vi "Do Action.vi"(7 "Self Enqueuer":refnum<class "Message Enqueuer.lvclass">, 8 "error in (no error)":errorcluster, 11 "Show Assert in":refnum<class "Show Assert.lvclass">) -> (0 "error out":errorcluster)   [LabVIEW 2016, in "Assert API Components.lvlib" / "Assert Display.lvlib" / "Main Display.lvlib" / "Show Assert.lvclass"]
uses:
  Show Assert.lvclass
  <vilib>/ActorFramework/Message Enqueuer/Message Enqueuer.lvclass
  <vilib>/Utility/traverseref.llb/TRef TravTarget.ctl
  Show Assert.lvclass/Show Assert.ctl
  Assert API Components/Assert API Components.lvlib
  <vilib>/Utility/traverseref.llb/VI Scripting - Traverse.lvlib
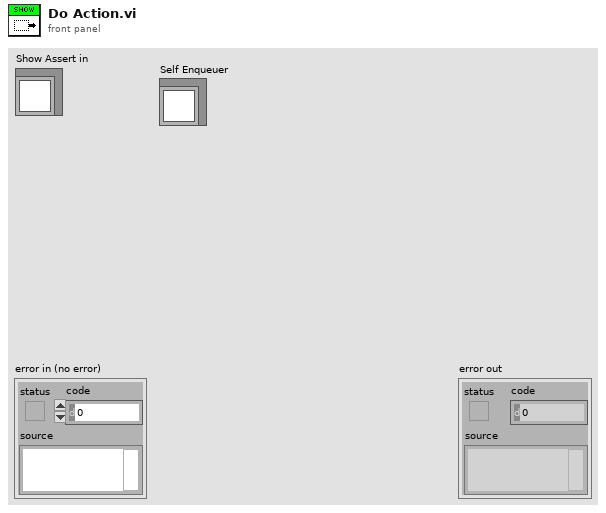
[diagram p1: front panel]
types:
  T1 = typedef "TRef TravTarget.ctl" = enum16{"FP", "BD", "Other"}
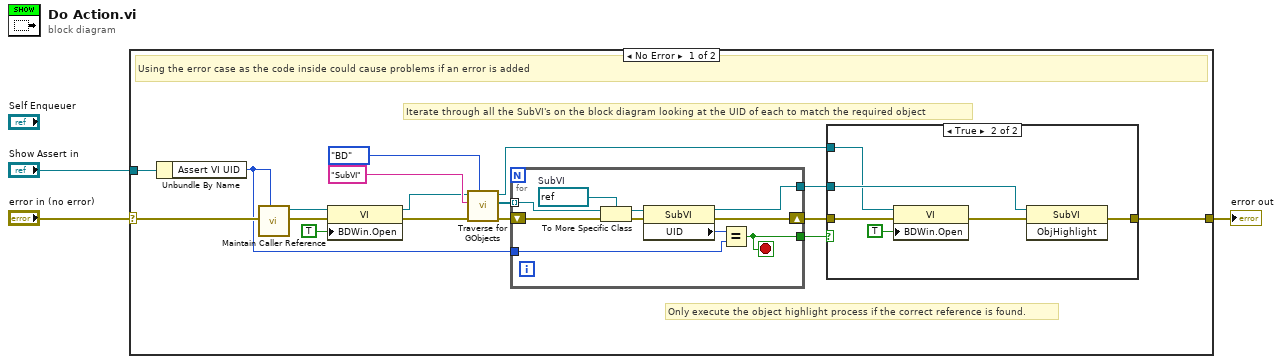
[diagram p0: block diagram]
diagram:
  n1 = case shown="No Error" "error in (no error)" {
    selector: "error in (no error)" -> [w19 w37]
    tunnel: "Show Assert in" -> [w18 _]
    tunnel: [w4 w37] -> w1
    frame No Error {
      # "Only execute the object highlight process if the correct reference is found."
      # "Iterate through all the SubVI's on the block diagram looking at the UID of each to match the required object"
      # "Using the error case as the code inside could cause problems if an error is added"
      n2 = Unbundle By Name(w18) -> ("Assert VI UID"=w5:i32)
      n3 = call "Maintain Caller Reference.vi"("UID"=w5) -> ("VI out"=w17:refnum<vi>)  [unwired: 10 in]
      n4 = property class="VI"(reference=w17, error in=w19, "BDWin.Open"=TRUE ("Block Diagram Window:Open")) -> (reference out=w7:refnum<vi>, error out=w6:errorcluster)
      n5 = call <vilib>:"Traverse for GObjects.vi"("Traverse Target"=TRef_TravTarget."BD", "error in (no error)"=w6, "Class Name"="SubVI", "VI Refnum"=w7) -> ("error out"=w13:errorcluster, "References"=w14:refnum<vi>[], "dup VI Refnum"=w15:refnum<vi>)  [unwired: 4 in, 1 out]
      n6 = for {
        tunnel: w14 -> [w29] mode=indexing
        tunnel: w5 -> [w35]
        tunnel: [w34] -> w12
        tunnel: [w33] -> w11
        shift-right: [w32] -> w10
        shift-left: w13 -> [w31]
        stop <- w34 stop-if-true
        w27 = refnum<vi> refnum  # SubVI
        n7 = To More Specific Class(target class=w27, reference=w29, error in=w31) -> (specific class reference=w28:refnum<vi>, error out=w30:errorcluster)
        n8 = property class="SubVI"(reference=w28, error in=w30) -> (reference out=w33:refnum<vi>, error out=w32:errorcluster, "UID"=w36:i32)
        n9 = Equal?(x=w36, y=w35) -> (x = y?=w34:bool)
      }
      n10 = case shown="True" w12 {
        tunnel: w11 -> [_ w26]
        tunnel: w10 -> [w20 w22]
        tunnel: [w20 w25] -> w4
        tunnel: w15 -> [_ w24]
        frame False {
        }
        frame True {
          n11 = property class="VI"(reference=w24, error in=w22, "BDWin.Open"=TRUE ("Block Diagram Window:Open")) -> (error out=w21:errorcluster)  [unwired: 1 out]
          n12 = invoke class="SubVI" method="ObjHighlight"(reference=w26, error in=w21) -> (error out=w25:errorcluster)  [unwired: 1 in, 2 out]
        }
      }
    }
    frame Error {
    }
  }
  "error out" <- w1
